vi "PH_PSDBWriter.write PSDB.vi"(0 "VI in":refnum<vi>, 5 "error in":errorcluster) -> (14 "VI out":refnum<vi>, 16 "PSDB Error code":i32, 17 "Data Status":T1 items=["no info", "no Data collection", "no problem", "Error getting the ID", "Error writing Data", "Error getting the subsystem", "Error getting the Shot ID", "Error getting the Shot Types", "Error getting the Experiments", "Error verifying wanted Shottype", "Error verifying wanted Experiment"], 19 "error out":errorcluster)   [LabVIEW 2014, in "PH_PSDBWriter.lvlib"]
uses:
  PH_PSDBWriter.lvlib
  PH_PSDBWriter.Data Status.ctl
  PH_Common/PH_Common.lvlib
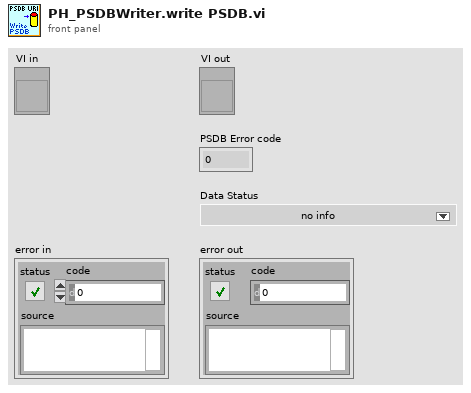
[diagram p1: front panel]
types:
  T1 = typedef "PH_PSDBWriter.lvlib/PH_PSDBWriter.Data Status.ctl" = i16
  T2 = typedef "PH_PSDBWriter.lvlib/PH_PSDBWriter.i attribute.ctl" = cluster{"PSDB Status Service ID":i32, "Instance ID":i32, "Shot #":i32, "Subsystem":T3, "Data Status":T1, "Ref PSDB Status":refnum<vi>, "PSDB Error Code":i32, "PSDB Dataset":T4, "PSDB Thread":cluster{"Ref":refnum<vi>, "Q-Ref":refnum<queue>}, "PSDB Credentials":T12}
  T3 = typedef "PH_PSDBWriter.lvlib/PH_PSDBWriter.PHELIX-Subsystems.ctl" = i32
  T4 = typedef "PH_PSDBWriter.lvlib/PH_PSDBWriter.PSDB Dataset.ctl" = cluster{"Version":i32, "2D data Input":T5[], "Boolean Input":T7[], "Image Input":T8[], "Numeric Input":T10[], "String Input":T11[]}
  T5 = typedef "PH_PSDBWriter.lvlib/PH_PSDBWriter.2D dataset.ctl" = cluster{"name":string, "data":dbl[][], "axis description":T6}
  T6 = typedef "PSDB.lvlib/PSDB_AxisDescription.ctl" = cluster{"x axis label":string, "y axis label":string, "x axis unit":string, "y axis unit":string}
  T7 = typedef "PH_PSDBWriter.lvlib/PH_PSDBWriter.Boolean dataset.ctl" = cluster{"name":string, "data":bool, "unit":string}
  T8 = typedef "PH_PSDBWriter.lvlib/PH_PSDBWriter.Image dataset.ctl" = cluster{"name":string, "data":T9, "unit":string}
  T9 = typedef "IMAQ Image.ctl" = refnum<image>
  T10 = typedef "PH_PSDBWriter.lvlib/PH_PSDBWriter.Numeric dataset.ctl" = cluster{"name":string, "data":dbl, "unit":string}
  T11 = typedef "PH_PSDBWriter.lvlib/PH_PSDBWriter.String dataset.ctl" = cluster{"name":string, "data":string, "unit":string}
  T12 = typedef "PH_Common.lvlib/PH_Connection.PSDB Credentials.ctl" = cluster{"PW":string, "ID":string, "DS":string}
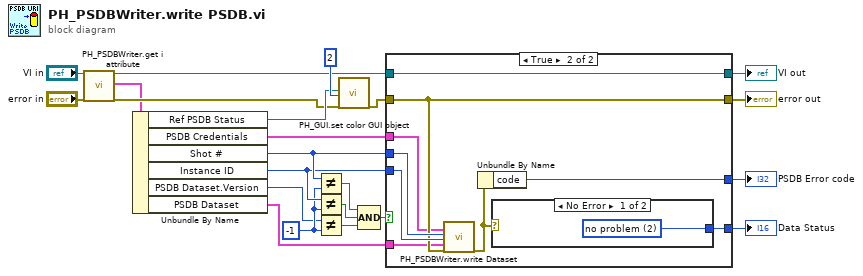
[diagram p0: block diagram]
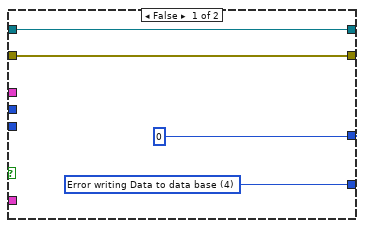
[diagram p2: hidden frame]
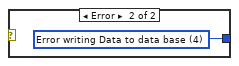
[diagram p3: hidden frame]
diagram:
  w4 = -1 ("y")
  n1 = call "PH_PSDBWriter.get i attribute.vi"("i ref in"="VI in", "error in (no error)"="error in") -> ("i ref out"=w5:refnum<vi>, "i attribute"=w8:T2, "error out"=w19:errorcluster)  [unwired: 15 in]
  n2 = Unbundle By Name(w8) -> ("Ref PSDB Status"=w21:refnum<vi>, "PSDB Credentials"=w1:T12, "Shot #"=w10:i32, "Instance ID"=w9:i32, "PSDB Dataset.Version"=w3:i32, "PSDB Dataset"=w17:T4)
  n3 = Not Equal?(x=w10, y=w4) -> (x != y?=w13:bool)
  n4 = Not Equal?(x=w9, y=w4) -> (x != y?=w14:bool)
  n5 = Not Equal?(x=w3, y=w4) -> (x != y?=w15:bool)
  n6 = call "PH_GUI.set color GUI object.vi"("GUI object Ref"=w21, "State"=2, "error in (no error)"=w19) -> ("error out"=w20:errorcluster)  [unwired: 16 in]
  n7 = Compound Arithmetic op=AND(w13, w14, w15) -> (w2:bool)
  n8 = case shown="True" w2 {
    tunnel: w20 -> [w24 w29]
    tunnel: w9 -> [_ w35]
    tunnel: w17 -> [_ w28]
    tunnel: [w26 w34] -> w12
    tunnel: w5 -> [w25 w32]
    tunnel: [w25 w32] -> w18
    tunnel: [w24 w29] -> w11
    tunnel: w10 -> [_ w33]
    tunnel: [0 ("code") w30] -> w16
    tunnel: w1 -> [_ w27]
    frame False {
      w26 = T1 4 items=["no info", "no Data collection", "no problem", "Error getting the instance ID", "Error writing Data to data base", "Error concerning the subsystem"] ("Data Status")
    }
    frame True {
      n9 = call "PH_PSDBWriter.write Dataset.vi"("PSDB Credentials"=w27, "Shot #"=w33, "Instance ID"=w35, "Data to write to PSDB"=w28, "error in (no error)"=w29) -> ("error out"=w31:errorcluster)  [unwired: 14 in]
      n10 = Unbundle By Name(w31) -> ("code"=w30:i32)
      n11 = case shown="No Error" w31 {
        tunnel: [w36 w37] -> w34
        frame No Error {
          w36 = T1 2 items=["no info", "no Data collection", "no problem", "Error getting the instance ID", "Error writing Data to data base", "Error concerning the subsystem"] ("Data Status")
        }
        frame Error {
          w37 = T1 4 items=["no info", "no Data collection", "no problem", "Error getting the instance ID", "Error writing Data to data base", "Error concerning the subsystem"] ("Data Status")
        }
      }
    }
  }
  "VI out" <- w18
  "PSDB Error code" <- w16
  "Data Status" <- w12
  "error out" <- w11
